vi "GET Output Voltage Limits.vi"() -> (0 "Minimum Output Voltage":dbl, 1 "Maximum Output Voltage":dbl)   [LabVIEW 2013]
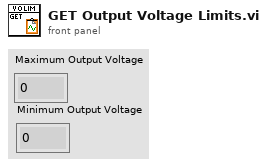
[diagram p1: front panel]
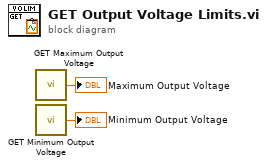
[diagram p0: block diagram]
diagram:
  n1 = call "GET Maximum Output Voltage.vi"() -> ("Maximum Output Voltage"=→"Maximum Output Voltage":dbl)
  n2 = call "GET Minimum Output Voltage.vi"() -> ("Minimum Output Voltage"=→"Minimum Output Voltage":dbl)
